vi "Get Channel Names.vi"(8 "error in (no error)":errorcluster, 11 "Electrophysiology in":refnum<class "Electrophysiology.lvclass">) -> (0 "error out":errorcluster, 2 "Strings and Numbers":cluster{refnum<k21>, i32}[](array[cluster]), 3 "Electrophysiology out":refnum<class "Electrophysiology.lvclass">)   [LabVIEW 2012, in "AcquisitionCoreObjects.lvlib" / "Electrophysiology.lvclass"]
uses:
  Electrophysiology.lvclass
  <resource>/objmgr/daqmx.rc
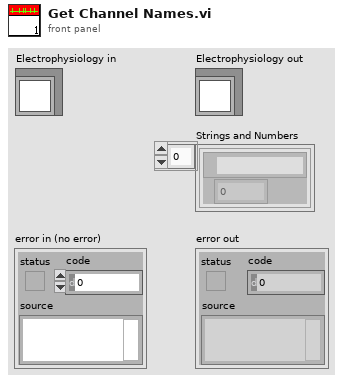
[diagram p1: front panel]
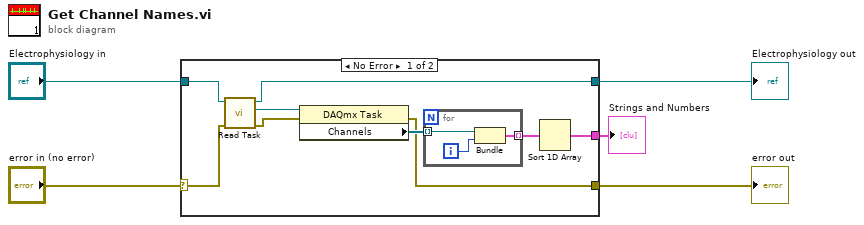
[diagram p0: block diagram]
diagram:
  n1 = case shown="No Error" "error in (no error)" {
    selector: "error in (no error)" -> [w9 w19]
    tunnel: [w7 w19] -> w4
    tunnel: [w10 w18] -> w2
    tunnel: "Electrophysiology in" -> [w11 w18]
    tunnel: [w6 _] -> w1
    frame No Error {
      n2 = call-dynamic "Read Task.vi"("error in (no error)"=w9, "AcquireTraces in"=w11) -> ("error out"=w8:errorcluster, "Task"=w12:refnum<k21>, "AcquireTraces out"=w10:refnum<class "Electrophysiology.lvclass">)  [unwired: 7 in]
      n3 = property class="DAQmx Task"(reference=w12, error in=w8) -> (error out=w7:errorcluster, "Channels"=w14:refnum<k21>[])  [unwired: 1 out]
      n4 = for {
        tunnel: w14 -> [w17] mode=indexing
        tunnel: [w16] -> w13 mode=indexing
        i -> [w15]
        n5 = Bundle(w17, w15) -> (w16:cluster{refnum<k21>, i32})  [unwired: 1 in]
      }
      n6 = Sort 1D Array(array=w13) -> (sorted array=w6:cluster{refnum<k21>, i32}[])
    }
    frame Error {
    }
  }
  "error out" <- w4
  "Electrophysiology out" <- w2
  "Strings and Numbers" <- w1
